vi "RunSaveImagesExperiment.vi"(11 "Save raw data":bool) -> ()   [LabVIEW 2011]
uses:
  Camera/CIGrabControlMsg.ctl
  Camera/CIGrabControlMsgEnum.ctl
  Camera/CIGrabParams.ctl
  qtrk/QTrk.llb/QTrkInstance.ctl
  Typedefs/TrackingConfigType.ctl
  qtrk/QTrk.llb/QTrkLocalizationType.ctl
  qtrk/QTrk.llb/QTrkZCommandType.ctl
  qtrk/QTrk.llb/ResultManagerInstance.ctl
  Typedefs/CmdData_NewFrame.ctl
  <vilib>/vision/Image Controls.llb/IMAQ Image.ctl
  Typedefs/CmdEnum_CameraFrameType.ctl
  ExperimentProgram/ExProgCommandEnumType.ctl
  GlobalVariables.vi
panel:
  out "Image saving speed\n(img/s)":dbl
  out "Number of queued images":i32
  out "Instruction index":i32
  out "Frame #":i32
  in  "Stop experiment":bool
  out "End grabbing loop":bool
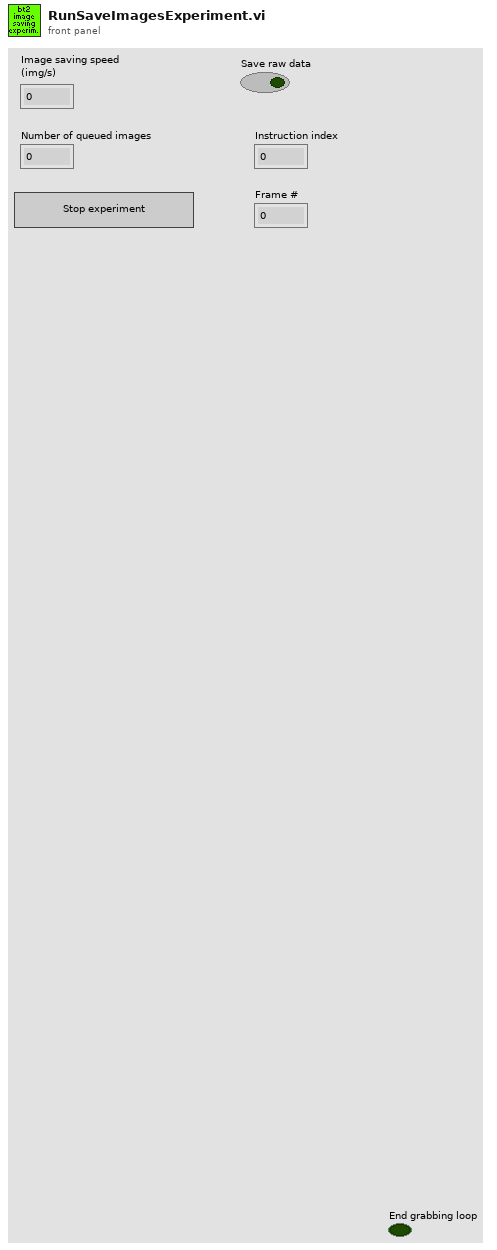
[diagram p1: front panel]
types:
  T1 = typedef "CIGrabControlMsg.ctl" = cluster{"Msg":T2}
  T2 = typedef "CIGrabControlMsgEnum.ctl" = enum16{"Stop", "EnableTracking", "DisableTracking"}
  T3 = typedef "CIGrabParams.ctl" = cluster{"Corner-based bead pos (out)":cluster{"X":i32, "Y":i32}[], "QTrk Instance":T4, "Tracking Config":T5, "ResultManager":T8, "Send to queue?":bool}
  T4 = typedef "QTrkInstance.ctl" = cluster{"QTrk Pointer":u64}
  T5 = typedef "TrackingConfigType.ctl" = cluster{"Number of steps":i32, "ZLUT stepsize (um)":sgl, "Z correction factor":sgl, "Start piezo Z (um)":sgl, "Pixel size (nm)":sgl, "2D Localization Type":T6, "Z Command (None)":T7, "Z Piezo scale":bool}
  T6 = typedef "QTrkLocalizationType.ctl" = enum16{"Center-of-Mass", "1D Cross-Correlation", "Quadrant Interpolation", "Gaussian 2D MLE", "QI + ZLUTAlign", "ZLUTAlign"}
  T7 = typedef "QTrkZCommandType.ctl" = enum16{"Nothing", "ComputeZ", "BuildRadialZLUT", "BuildImageZLUT", "RadialZLUT+ImageZLUT"}
  T8 = typedef "ResultManagerInstance.ctl" = cluster{"InstancePtr":u64}
  T9 = typedef "CmdData_NewFrame.ctl" = cluster{"Buffer Image":T10, "Frame #":i32, "Hardware ROI Index":i32, "Timestamp":dbl, "Type":T11}
  T10 = typedef "IMAQ Image.ctl" = refnum<image>
  T11 = typedef "CmdEnum_CameraFrameType.ctl" = enum16{"Full", "HardwareROI", "EndGrabMarker"}
  T12 = typedef "ExProgCommandEnumType.ctl" = enum16{"wait", "move", "acquire", "idle", "rmove", "when", "section", "stop"}
  T13 = typedef "CameraInstance.ctl" = cluster{"VI refs":T14, "Camera state":variant}
  T14 = typedef "CameraInterface.ctl" = cluster{"Close":T15, "Get/Set generic config":T16, "Grab":T17, "Show Settings Dialog":T18, "AdjustBeadPos":T19, "Save/load camera settings":T20}
  T15 = typedef "CICloseType.ctl" = refnum<vi>
  T16 = typedef "CIGetSetGenericConfig.ctl" = refnum<vi>
  T17 = typedef "CIGrabType.ctl" = refnum<vi>
  T18 = typedef "CISettingsDlg.ctl" = refnum<vi>
  T19 = typedef "CIAdjustBeadPos.ctl" = refnum<vi>
  T20 = typedef "CISaveLoadSettings.ctl" = refnum<vi>
  T21 = typedef "MeasureConfigType.ctl" = cluster{"Bead locations":cluster{"X":i32, "Y":i32}[], "ROI":i32, "Experiment base path":path, "Image output subdir":string, "Output mode":T22, "Traces output subdir":string, "QTrk Settings":T23, "Tracking Config":T5, "Experiment Name":string, "Program":T24, "ZLUT":sgl[][][], "Camera settings":T30, "Experiment Script":string, "Max frames in memory":i32, "Save traces as binary":bool, "Pixel Calibration Gain Image":string, "Pixel Calibration Offset Image":string, "Use pixel calibration images":bool, "Internal camera settings":string}
  T22 = typedef "MeasureConfigOutputMode.ctl" = enum16{"None", "Track", "SaveImages"}
  T23 = typedef "QTrkSettings.ctl" = cluster{"Image width":i32, "Image height":i32, "Number of threads (CPU based)":i32, "CUDA Device":i32, "COM Background correction factor":sgl, "ZLUT MinRadius":sgl, "ZLUT Radial sample density":sgl, "ZLUT Angular sample density":sgl, "ZLUT ROI Coverage":sgl, "QI Iterations":i32, "QI MinRadius":sgl, "QI Radial sample density":sgl, "QI Angular sample density":sgl, "QI ROI Coverage":sgl, "QI Angular Step \nIteration Factor":sgl, "XCOR Profile Length":i32, "XCOR Profile Width":i32, "XCOR Iterations":i32, "Gaussian 2D Fit Iterations":i32, "Gaussian 2D Sigma (pixels)":sgl}
  T24 = typedef "ExperimentProgramType.ctl" = cluster{"Commands":T25[], "Motor Axis accuracy conditions":T27, "Axis flags":T29}
  T25 = typedef "ExProgCommandType.ctl" = cluster{"cmd":T12, "axis":T26, "value/pos":dbl, "speed":dbl, "name":string}
  T26 = typedef "MotorAxisEnum.ctl" = enum16{"no axis", "magrot", "magpos", "px", "py", "pz", "camx", "camy"}
  T27 = typedef "MotorPosType.ctl" = cluster{"Magnet Z":dbl, "Magnet rotation":dbl, "Camera":T28, "Piezo XY":T28, "Piezo Z":dbl}
  T28 = typedef "XYf.ctl" = cluster{"X":sgl, "Y":sgl}
  T29 = typedef "MotorPosFlagsType.ctl" = cluster{"Magnet Z":bool, "Magnet rotation":bool, "Camera":cluster{"X":bool, "Y":bool}, "Piezo XY":cluster{"X":bool, "Y":bool}, "Piezo Z":bool}
  T30 = typedef "GenericCameraConfigType.ctl" = cluster{"Framerate (Hz)":i32, "Exposure time (us)":i32, "Image size":cluster{"Width":i32, "Height":i32}, "Number of buffers":i32}
  T31 = typedef "ExProgState.ctl" = cluster{"Wanted Motorpos":T27, "Goal motorpos":T27, "Instruction":i32, "Speed":T27, "New instruction?":bool, "Instruction start time":dbl}
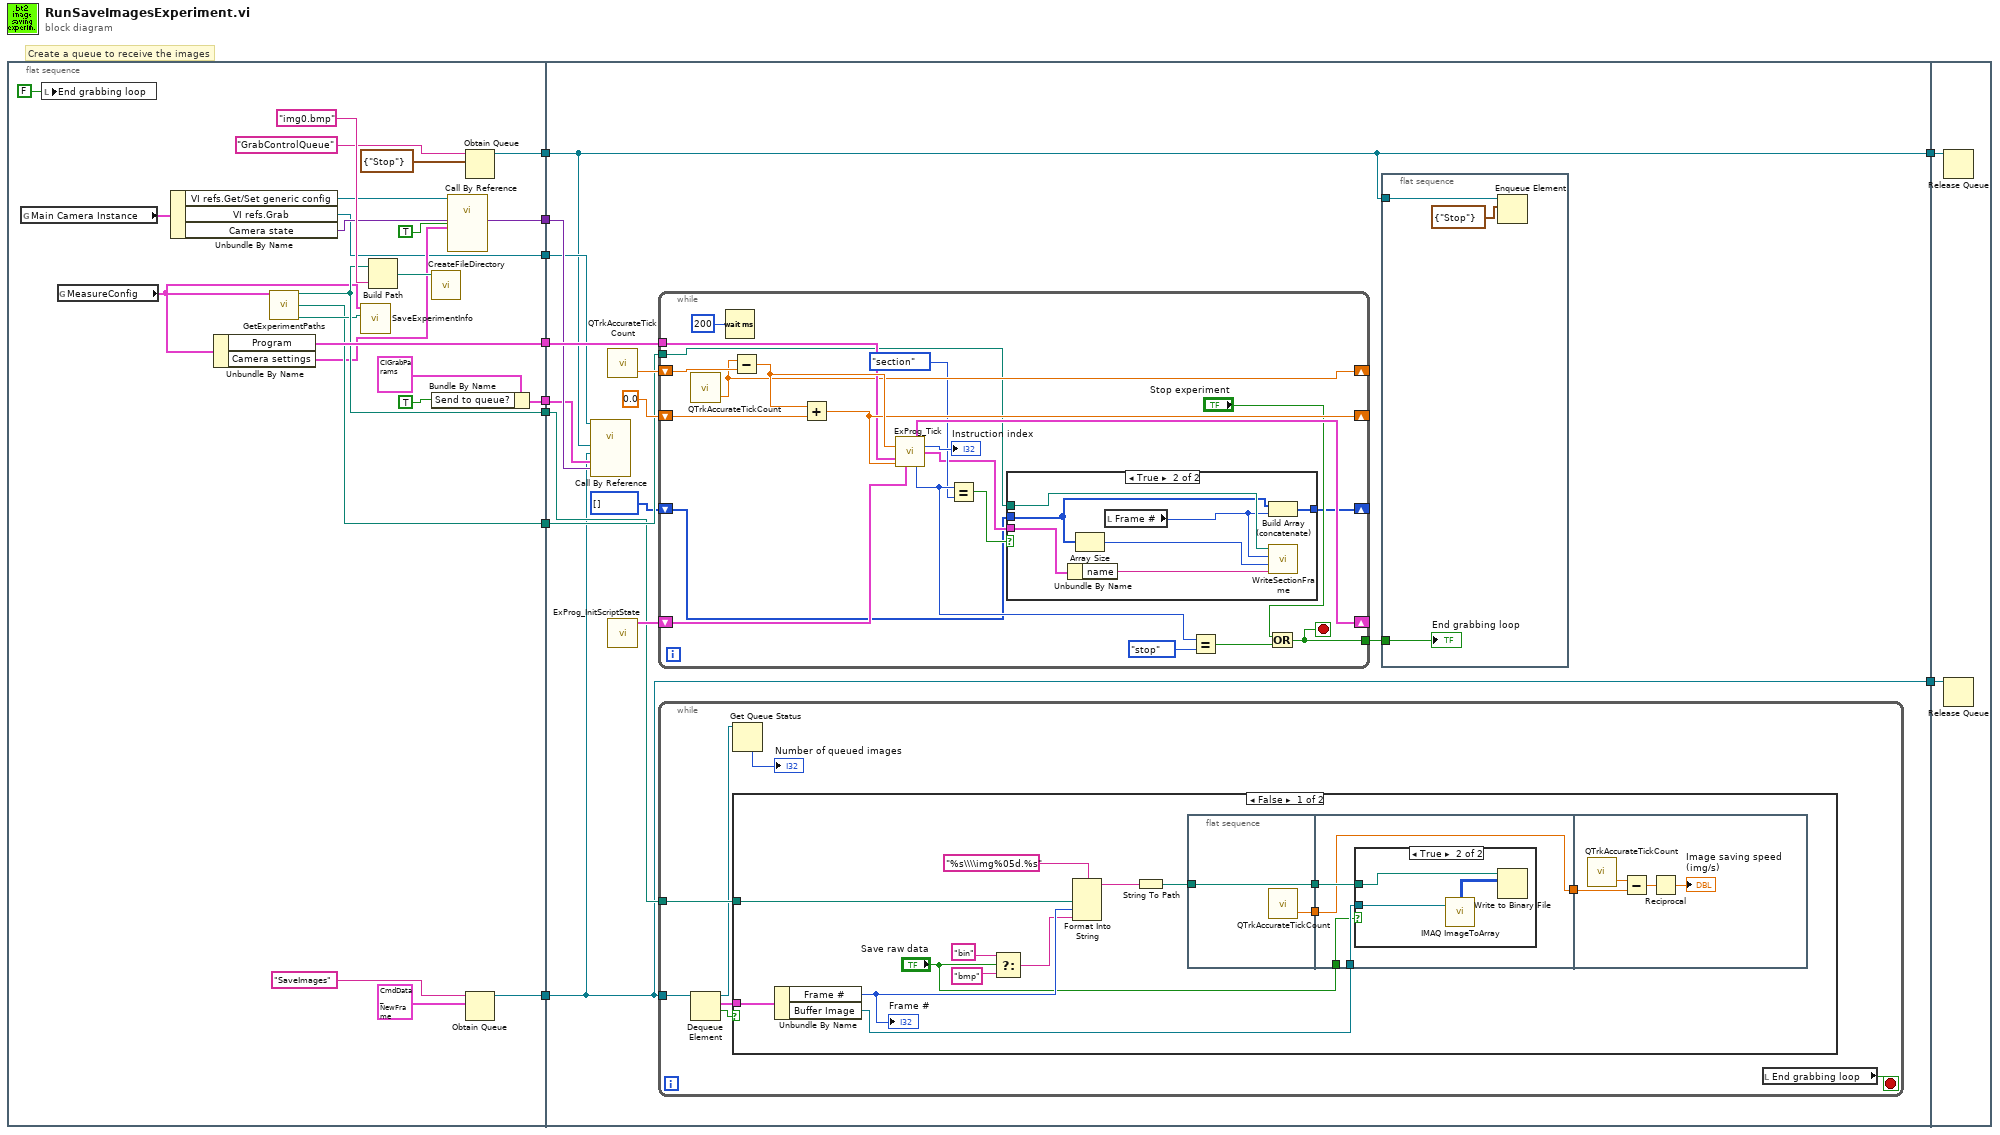
[diagram p0: block diagram]
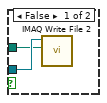
[diagram p2: hidden frame]
diagram:
  # "Create a queue to receive the images"
  n1 = flat-sequence {
    tunnel: [w28] -> w10
    tunnel: [w32] -> w8
    tunnel: [w29] -> w7
    tunnel: [w24] -> w6
    tunnel: [w18] -> w5
    tunnel: [w15] -> w4
    tunnel: [w12] -> w3
    tunnel: [w11] -> w2
    tunnel: w10 -> [w37]
    tunnel: [w37] -> w9
    tunnel: w8 -> [w45]
    tunnel: w7 -> [w40]
    tunnel: w6 -> [w42]
    tunnel: w5 -> [w39]
    tunnel: w4 -> [w38]
    tunnel: w3 -> [w35]
    tunnel: w2 -> [w36]
    tunnel: [w35] -> w1
    tunnel: w9 -> [w116]
    tunnel: w1 -> [w117]
    frame #0 {
      n2 = global read "GlobalVariables.vi" "Main Camera Instance"() -> (w23:T13)
      n3 = local write "End grabbing loop"(FALSE ("End grabbing loop")) -> ()
      n4 = global read "GlobalVariables.vi" "MeasureConfig"() -> (w25:T21)
      n5 = Unbundle By Name(w23) -> ("VI refs.Get/Set generic config"=w22:T16, "VI refs.Grab"=w11:T17, "Camera state"=w19:variant)
      n6 = Unbundle By Name(w25) -> ("Program"=w32:T24, "Camera settings"=w20:T30)
      n7 = call "GetExperimentPaths.vi"("MeasureConfig"=w25) -> ("[base]\\images\\[expname]\\"=w29:path, "[base]\\traces\\[expname]_sections.txt"=w24:path, "[base]\\traces\\[expname]_info.txt"=w26:path)  [unwired: 6 in, 6 out]
      n8 = call "SaveExperimentInfo.vi"("File path"=w26, "MeasureConfig"=w25) -> ()  [unwired: 10 in]
      n9 = Build Path(base path=w29, name or relative path="img0.bmp") -> (appended path=w31:path)
      n10 = call "CreateFileDirectory.vi"("filename"=w31) -> ()  [unwired: 10 in, 1 out]
      n11 = Bundle By Name(cluster=T3 {"Corner-based bead pos (out)"=[], "QTrk Instance"={"QTrk Pointer"=0}, "Tracking Config"={"Number of steps"=0, "ZLUT stepsize (um)"=0.0, "Z correction factor"=0.0, "Start piezo Z (um)"=0.0, "Pixel size (nm)"=0.0, "2D Localization Type"=enum."Quadrant Interpolation", "Z Command (None)"=enum."Nothing", "Z Piezo scale"=FALSE}, "ResultManager"={"InstancePtr"=0}, "Send to queue?"=TRUE} ("TrackingParameters"), "Send to queue?"=TRUE) -> (w15:T3)
      n12 = call-by-ref "?"(reference=w22, "Set? (F)"=TRUE, "GenericCameraConfig"=w20, "Camera state"=w19) -> ("Camera state (out)"=w18:variant)  [unwired: 8 in, 3 out]
      n13 = Obtain Queue(name (unnamed)="GrabControlQueue", element data type=T1 {"Msg"=enum."Stop"} ("GrabControlMsg")) -> (queue out=w12:refnum<queue>)  [unwired: 3 in, 2 out]
      n14 = Obtain Queue(name (unnamed)="SaveImages", element data type=T9 {"Buffer Image"=refnum, "Frame #"=0, "Hardware ROI Index"=0, "Timestamp"=0.0, "Type"=enum."Full"} ("Cluster")) -> (queue out=w28:refnum<queue>)  [unwired: 3 in, 2 out]
    }
    frame #1 {
      n15 = call-by-ref "?"(reference=w36, "Camera data"=w39, "TrackingParameters"=w38, "Output Queue"=w37, "GrabControlQueue"=w35) -> ()  [unwired: 8 in, 3 out]
      n16 = call "QTrkAccurateTickCount.vi"() -> ("seconds"=w47:dbl)  [unwired: 2 in, 1 out]
      n17 = call "ExProg_InitScriptState.vi"() -> ("Script exec state out"=w44:T31)  [unwired: 11 in]
      n18 = while {
        shift-right: [w104] -> _
        shift-left: 0.0 ("y") -> [w105]
        tunnel: w45 -> [w103]
        shift-right: [w100] -> _
        shift-left: w44 -> [w102]
        shift-right: [w101] -> _
        shift-left: w47 -> [w107]
        tunnel: [w97] -> w43
        tunnel: w42 -> [w89]
        shift-right: [w87] -> _
        shift-left: i32[] [] ("initialized array") -> [w88]
        stop <- w97 stop-if-true
        n19 = call "QTrkAccurateTickCount.vi"() -> ("seconds"=w101:dbl)  [unwired: 2 in, 1 out]
        n20 = Wait (ms)(milliseconds to wait=u32 200) -> ()  [unwired: 1 out]
        n21 = Subtract(x=w101, y=w107) -> (x-y=w106:dbl)
        n22 = Add(x=w106, y=w105) -> (x+y=w104:dbl)
        n23 = call "ExProg_Tick.vi"("Timestep (s)"=w106, "Program"=w103, "Current time (s)"=w104, "Script exec state in"=w102) -> ("Script exec state out"=w100:T31, "Instruction index"=→"Instruction index":i32, "Last instruction"=w90:T25, "Last command"=w93:T12)  [unwired: 7 in, 1 out]
        n24 = Equal?(x=w93, y=ExProgCommandEnumType."section") -> (x = y?=w91:bool)
        n25 = case shown="True" w91 {
          tunnel: w88 -> [w108 w113]
          tunnel: [w108 w115] -> w87
          tunnel: w89 -> [_ w114]
          tunnel: w90 -> [_ w110]
          frame False {
          }
          frame True {
            n26 = Unbundle By Name(w110) -> ("name"=w111:string)
            n27 = Array Size(array=w113) -> (size(s)=w112:i32)
            n28 = local read "Frame #"() -> (w109:i32)
            n29 = Build Array (concatenate)(w113, w109) -> (w115:i32[])
            n30 = call "WriteSectionFrame.vi"("section name"=w111, "section index"=w112, "section frame"=w109, "[base]\\traces\\[expname]_sections.txt"=w114) -> ()  [unwired: 8 in]
          }
        }
        n31 = Equal?(x=w93, y=ExProgCommandEnumType."stop") -> (x = y?=w98:bool)
        n32 = Or(x="Stop experiment", y=w98) -> (x .or. y?=w97:bool)
      }
      n33 = while {
        tunnel: w37 -> [w57]
        tunnel: w40 -> [w54]
        stop <- w53 stop-if-true
        n34 = Dequeue Element(queue=w57) -> (queue out=w51:refnum<queue>, element=w55:T9, timed out?=w56:bool)  [unwired: 2 in, 1 out]
        n35 = Get Queue Status(queue=w51) -> (# elements in queue=→"Number of queued images":i32)  [unwired: 2 in, 7 out]
        n36 = case shown="False" w56 {
          tunnel: w55 -> [w71 _]
          tunnel: w54 -> [w68 _]
          frame False {
            n37 = Unbundle By Name(w71) -> ("Frame #"=w67:i32, "Buffer Image"=w70:T10)
            "Frame #" <- w67
            n38 = Select(t="bin", s="Save raw data", f="bmp" ("input 3")) -> (s? t:f=w59:string)
            n39 = Format Into String(format string="%s\\\\img%05d.%s", w68, w67, w59) -> (resulting string=w66:string)  [unwired: 2 in, 1 out]
            n40 = String To Path(string=w66) -> (path=w65:path)
            n41 = flat-sequence {
              tunnel: w65 -> [w73]
              tunnel: [w73] -> w64
              tunnel: [w72] -> w63
              tunnel: w70 -> [w77]
              tunnel: w64 -> [w76]
              tunnel: w63 -> [w75]
              tunnel: [w75] -> w62
              tunnel: "Save raw data" -> [w74]
              tunnel: w62 -> [w85]
              frame #0 {
                n42 = call "QTrkAccurateTickCount.vi"() -> ("seconds"=w72:dbl)  [unwired: 2 in, 1 out]
              }
              frame #1 {
                n43 = case shown="True" w74 {
                  tunnel: w77 -> [w79 w82]
                  tunnel: w76 -> [w78 w81]
                  frame False {
                    n44 = call-poly "IMAQ Write File 2"("File Path"=w78, "Image"=w79) -> ()  [unwired: 8 in, 2 out]
                  }
                  frame True {
                    n45 = call "IMAQ ImageToArray"("Image"=w82) -> ("Image Pixels (U8)"=w80:u8[][])  [unwired: 3 in, 4 out]
                    n46 = Write to Binary File(file (use dialog)=w81, data=w80) -> ()  [unwired: 4 in, 3 out]
                  }
                }
              }
              frame #2 {
                n47 = call "QTrkAccurateTickCount.vi"() -> ("seconds"=w86:dbl)  [unwired: 2 in, 1 out]
                n48 = Subtract(x=w86, y=w85) -> (x-y=w84:dbl)
                n49 = Reciprocal(x=w84) -> (1/x=→"Image saving speed\n(img/s)":dbl)
              }
            }
          }
          frame True {
          }
        }
        n50 = local read "End grabbing loop"() -> (w53:bool)
      }
      n51 = flat-sequence {
        tunnel: w43 -> [w50]
        tunnel: w35 -> [w49]
        frame #0 {
          n52 = Enqueue Element(queue=w49, element=T1 {"Msg"=enum."Stop"}) -> ()  [unwired: 2 in, 3 out]
          "End grabbing loop" <- w50
        }
      }
    }
    frame #2 {
      n53 = Release Queue(queue=w117) -> ()  [unwired: 2 in, 3 out]
      n54 = Release Queue(queue=w116) -> ()  [unwired: 2 in, 3 out]
    }
  }
